vi "RTS DTR CTS monitor.vi"() -> ()   [LabVIEW 2013]
uses:
  <vilib>/Instr/_visa.llb/VISA Open Access Mode.ctl
  NanoArduino/NanoCmds.ctl
  Test Globals/Global 1.vi
panel:
  out "DTR":bool
  in  "Read DTR":bool
  out "RTS":bool
  in  "Read RTS":bool
  out "DTR State":i16(ring)=-1 items=["Unknown"=-1, "Unasserted"=0, "Asserted"=1]
  out "btw controller port out":refnum<visa-resource-name>
  in  "BTW test controller":refnum<visa-resource-name>="COM21"
  out "CTS":bool
  out "DSR State":i16(ring) items=["Unknown"=-1, "Unasserted"=0, "Asserted"=1]
  out "RI State":i16(ring) items=["Unknown"=-1, "Unasserted"=0, "Asserted"=1]
  out "DCD State":i16(ring) items=["Unknown"=-1, "Unasserted"=0, "Asserted"=1]
  out "CTS State":i16(ring) items=["Unknown"=-1, "Unasserted"=0, "Asserted"=1]
  out "RTS State":i16(ring)=-1 items=["Unknown"=-1, "Unasserted"=0, "Asserted"=1]
  in  "stop":bool
  out "Modem port":refnum<visa-resource-name>
  in  "Read CTS":bool
  in  "Set Clear DTR":bool
  in  "Set Clear RTS":bool
  in  "Open serial?":bool=TRUE
  in  "Access Mode":T1=1 items=["VISA Defaults"=0, "Exclusive Lock"=1, "Load Configured Settings"=4]
  in  "flow control (0:none)":u16(ring)=2 items=["None", "XON/XOFF", "RTS/CTS", "XON/XOFF & RTS/CTS", "DTR/DSR", "XON/XOFF & DTR/DSR"]
  in  "Baud":dbl=115200.0
  in  "VISA Refnum in":refnum<visa-resource-name>="COM30"
  out "error out":errorcluster={"status"=TRUE, "code"=-1073807302, "source"="Property Node (arg 1) in RTS DTR CTS monitor.vi"}
  in  "error in (no error)":errorcluster
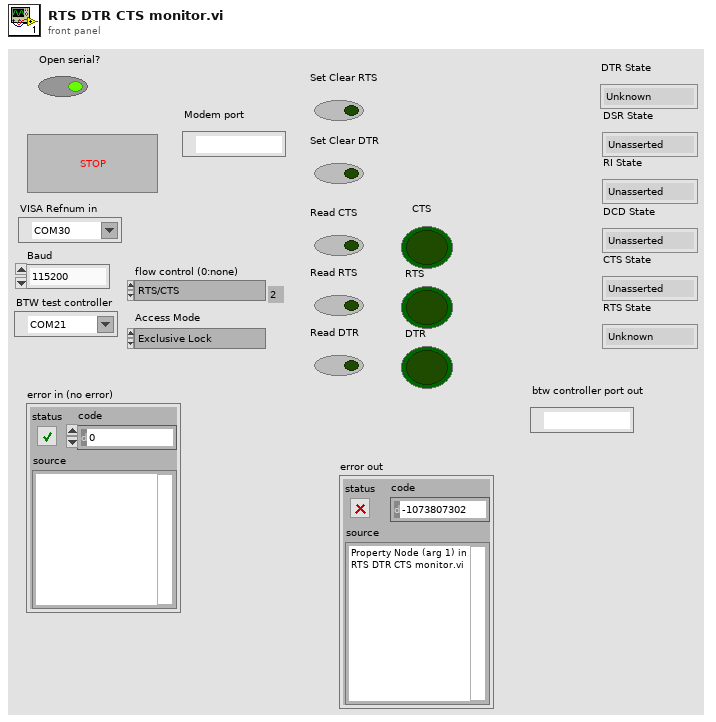
[diagram p1: front panel]
types:
  T1 = typedef "VISA Open Access Mode.ctl" = u32
  T2 = typedef "NanoCmds.ctl" = enum16{"Make digital port an output", "Make digital port an input", "Set digital pin high", "Set digital pin low", "Get digital pin state", "Get analog pin voltage", "Get analog pins difference", "Get ohms at analog pin", "Turn on current limit", "Reset Nano device", "Get digital pin state pullup", "Read current", "Initialize", "Power up uut", "Power down uut", "Get uut current draw", "Set ADC volts high", "Set ADC volts low", "Start up uut modem", "Get CTS state", "Get on_nsleep state", "Reset modem", "Get lid state", "Wait for lid closed", "Wait for lid open", "Power up, start, get curr", "Check if X2 shorted", "Power up and start up", "Check X3 shorted", "Get RTS state", "Get DTR state"}
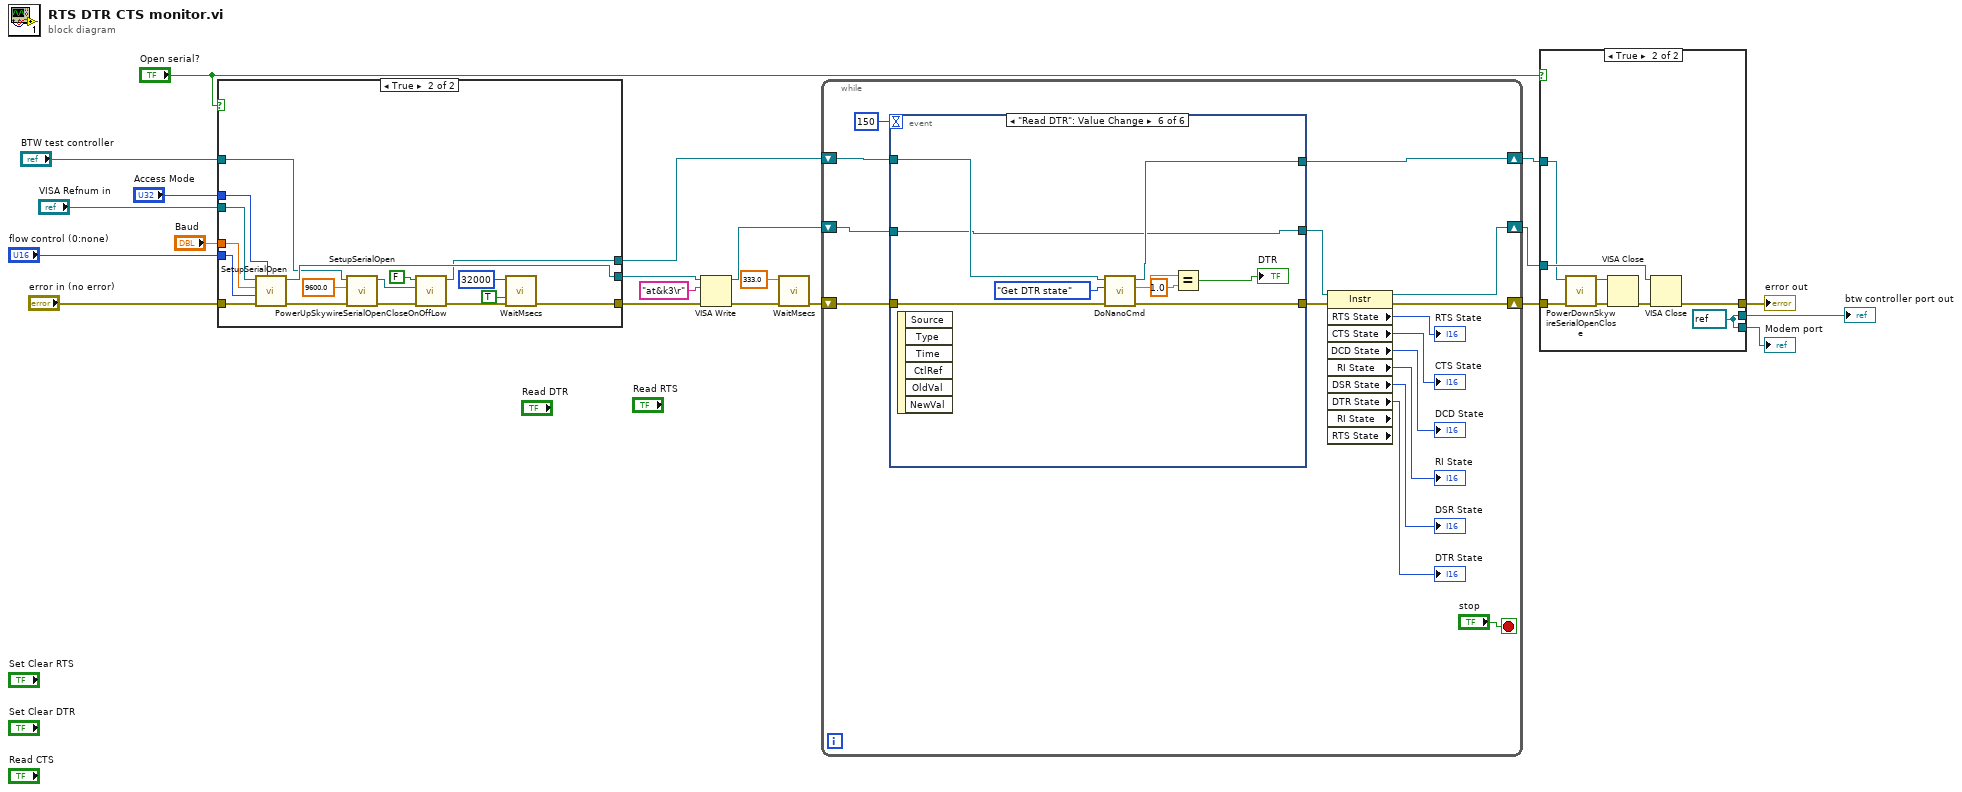
[diagram p0: block diagram]
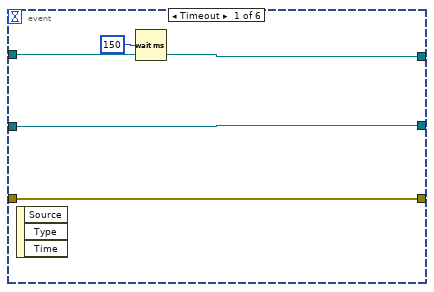
[diagram p3: hidden frame]
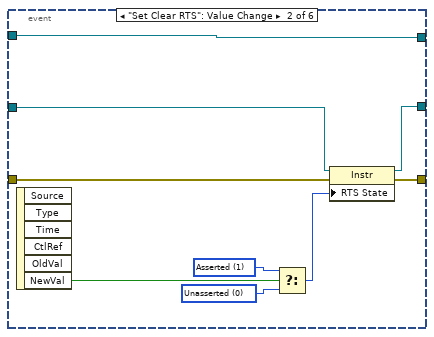
[diagram p4: hidden frame]
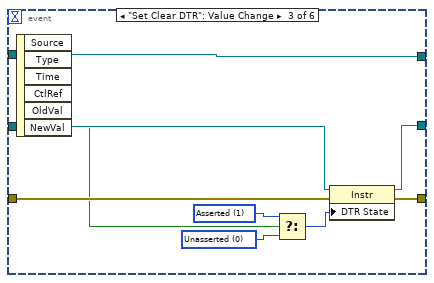
[diagram p5: hidden frame]
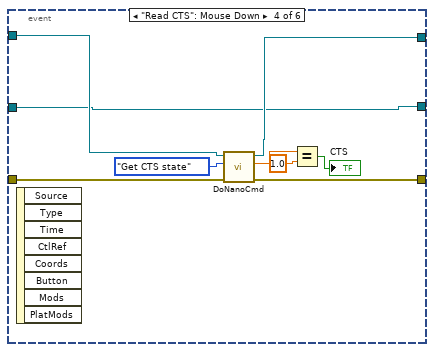
[diagram p6: hidden frame]
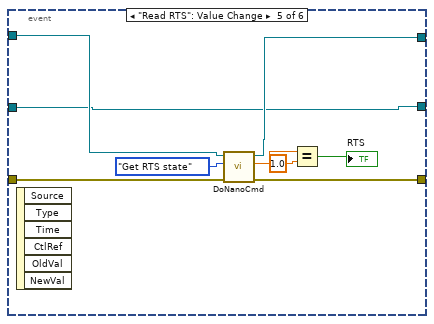
[diagram p7: hidden frame]
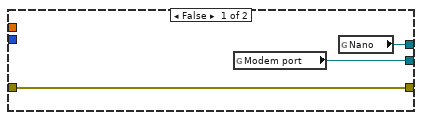
[diagram p8: hidden frame]
diagram:
  n1 = case shown="True" "Open serial?" {
    tunnel: "error in (no error)" -> [w24 w41]
    tunnel: [w24 w27] -> w15
    tunnel: "VISA Refnum in" -> [_ w40]
    tunnel: "Baud" -> [_ w39]
    tunnel: "flow control (0:none)" -> [_ w38]
    tunnel: "Access Mode" -> [_ w37]
    tunnel: [w23 w36] -> w16
    tunnel: [w22 w29] -> w3
    tunnel: "BTW test controller" -> [_ w34]
    frame False {
      n2 = global read "Global 1.vi" "Modem port"() -> (w23:refnum<visa-resource-name>)
      n3 = global read "Global 1.vi" "Nano"() -> (w22:refnum<visa-resource-name>)
    }
    frame True {
      n4 = call "SetupSerialOpen.vi"("Access Mode"=w37, "error in (no error)"=w41, "flow control (0:none)"=w38, "Baud"=w39, "VISA Refnum in"=w40) -> ("error out"=w35:errorcluster, "VISA session"=w36:refnum<visa-resource-name>)  [unwired: 5 in]
      n5 = call "SetupSerialOpen.vi"("error in (no error)"=w35, "Baud"=9600.0, "VISA Refnum in"=w34) -> ("error out"=w32:errorcluster, "VISA session"=w30:refnum<visa-resource-name>)  [unwired: 7 in]
      n6 = call "PowerUpSkywireSerialOpenCloseOnOffLow.vi"("error in (no error)"=w32, "VISA Refnum in"=w30, "Open COM21? (y)"=FALSE ("Open COM21?")) -> ("error out"=w28:errorcluster, "VISA resource name out"=w29:refnum<visa-resource-name>)  [unwired: 7 in]
      n7 = call "WaitMsecs.vi"("error in (no error)"=w28, "Show progress bar?"=TRUE, "Wait Msecs"=u32 32000) -> ("error out"=w27:errorcluster)  [unwired: 8 in]
    }
  }
  n8 = VISA Write(VISA resource name=w16, write buffer="at&k3\r", error in (no error)=w15) -> (VISA resource name out=w12:refnum<visa-resource-name>, error out=w13:errorcluster)  [unwired: 1 out]
  n9 = call "WaitMsecs.vi"("error in (no error)"=w13, "Wait Msecs"=333.0) -> ("error out"=w11:errorcluster)  [unwired: 9 in]
  n10 = while {
    shift-right: [w52] -> w8
    shift-left: w12 -> [w57]
    shift-right: [w43] -> w6
    shift-left: w11 -> [w56]
    shift-right: [w45] -> w2
    shift-left: w3 -> [w46]
    stop <- "stop" stop-if-true
    n11 = event shown="[5] \"Read DTR\": Value Change" {
      selector: _ -> [_ _ _ _ _ _]
      dyn-events: _ -> [_ _ _ _ _ _]
      timeout: 150 -> [_ _ _ _ _ _]
      tunnel: w57 -> [w59 w69 w76 w80 w90 w99]
      tunnel: w56 -> [w60 w70 w75 w83 w93 w102]
      tunnel: [w60 w65 w73 w82 w92 w101] -> w44
      tunnel: [w59 w64 w77 w80 w90 w99] -> w53
      tunnel: w46 -> [w58 w63 w71 w84 w94 w103]
      tunnel: [w58 w63 w71 w81 w91 w100] -> w45
      event Timeout {
        n12 = event-data() -> ()  [unwired: 1 in, 3 out]
        n13 = Wait (ms)(milliseconds to wait=u32 150) -> ()  [unwired: 1 out]
      }
      event "Set Clear RTS": Value Change {
        w66 = i16 0 items=["Unknown"=-1, "Unasserted"=0, "Asserted"=1] ("Serial Settings:Modem Line Settings:Line DTR State")
        w67 = i16 1 items=["Unknown"=-1, "Unasserted"=0, "Asserted"=1] ("Serial Settings:Modem Line Settings:Line DTR State")
        n14 = event-data() -> ("NewVal"=w68:bool)  [unwired: 1 in, 5 out]
        n15 = Select(t=w67, s=w68, f=w66) -> (s? t:f=w62:i16)
        n16 = property class="Instr"(reference=w69, error in=w70, "RTS State"=w62) -> (reference out=w64:refnum<visa-resource-name>, error out=w65:errorcluster)
      }
      event "Set Clear DTR": Value Change {
        w78 = i16 0 items=["Unknown"=-1, "Unasserted"=0, "Asserted"=1] ("Serial Settings:Modem Line Settings:Line DTR State")
        w79 = i16 1 items=["Unknown"=-1, "Unasserted"=0, "Asserted"=1] ("Serial Settings:Modem Line Settings:Line DTR State")
        n17 = event-data() -> ("NewVal"=w74:bool)  [unwired: 1 in, 5 out]
        n18 = Select(t=w79, s=w74, f=w78) -> (s? t:f=w72:i16)
        n19 = property class="Instr"(reference=w76, error in=w75, "DTR State"=w72) -> (reference out=w77:refnum<visa-resource-name>, error out=w73:errorcluster)
      }
      event "Read CTS": Mouse Down {
        n20 = event-data() -> ()  [unwired: 1 in, 8 out]
        n21 = call "DoNanoCmd.vi"("error in (no error)"=w83, "Nano Op"=NanoCmds."Get CTS state", "VISA resource name"=w84) -> ("error out"=w82:errorcluster, "Read Value"=w86:dbl, "VISA resource name 2"=w81:refnum<visa-resource-name>)  [unwired: 5 in, 1 out]
        n22 = Equal?(x=w86, y=1.0) -> (x = y?=→"CTS":bool)
      }
      event "Read RTS": Value Change {
        n23 = event-data() -> ()  [unwired: 1 in, 6 out]
        n24 = call "DoNanoCmd.vi"("error in (no error)"=w93, "Nano Op"=NanoCmds."Get RTS state", "VISA resource name"=w94) -> ("error out"=w92:errorcluster, "Read Value"=w95:dbl, "VISA resource name 2"=w91:refnum<visa-resource-name>)  [unwired: 5 in, 1 out]
        n25 = Equal?(x=w95, y=1.0) -> (x = y?=→"RTS":bool)
      }
      event "Read DTR": Value Change {
        n26 = event-data() -> ()  [unwired: 1 in, 6 out]
        n27 = call "DoNanoCmd.vi"("error in (no error)"=w102, "Nano Op"=NanoCmds."Get DTR state", "VISA resource name"=w103) -> ("error out"=w101:errorcluster, "Read Value"=w104:dbl, "VISA resource name 2"=w100:refnum<visa-resource-name>)  [unwired: 5 in, 1 out]
        n28 = Equal?(x=w104, y=1.0) -> (x = y?=→"DTR":bool)
      }
    }
    n29 = property class="Instr" props=["RTS State", "CTS State", "DCD State", "RI State", "DSR State", "DTR State", "RI State", "RTS State"](reference=w53, error in=w44) -> (reference out=w52:refnum<visa-resource-name>, error out=w43:errorcluster, "RTS State"=→"RTS State":i16, "CTS State"=→"CTS State":i16, "DCD State"=→"DCD State":i16, "RI State"=→"RI State":i16, "DSR State"=→"DSR State":i16, "DTR State"=→"DTR State":i16)  [unwired: 2 out]
  }
  n30 = case shown="True" "Open serial?" {
    tunnel: w8 -> [w109 w117]
    tunnel: [w109 w113] -> w7
    tunnel: w6 -> [w108 w112]
    tunnel: [w108 w110] -> w5
    tunnel: w2 -> [w107 w116]
    tunnel: [w107 w113] -> w1
    frame False {
    }
    frame True {
      w113 = refnum<visa-resource-name> refnum ("VISA session")
      n31 = call "PowerDownSkywireSerialOpenClose.vi"("error in (no error)"=w112, "VISA resource name"=w116) -> ("error out"=w114:errorcluster, "VISA resource name out"=w115:refnum<visa-resource-name>)  [unwired: 7 in, 1 out]
      n32 = VISA Close(VISA resource name=w115, error in (no error)=w114) -> (error out=w111:errorcluster)
      n33 = VISA Close(VISA resource name=w117, error in (no error)=w111) -> (error out=w110:errorcluster)
    }
  }
  "error out" <- w5
  "Modem port" <- w7
  "btw controller port out" <- w1
